vi "AWG simple.vi"() -> ()   [LabVIEW 2015]
uses:
  <instrlib>/niFgen/niFgen.llb/niFgen Output Mode.ctl
  <instrlib>/niFgen/niFgen.llb/niFgen Create Waveform (WDT).vi
panel:
  in  "FGEN Gain":dbl=5.0
  in  "User Gain":dbl=10.0
  out "Sample Rate":dbl
  out "error out":errorcluster
  in  "Resource Name":refnum<k15>="ArbWaveformGen"
  in  "Load Saved Waveform":bool
  in  "Save Current Waveform":bool
  in  "Apply Changes":bool
  in  "stop":bool
  out "Waveform Chart 2":waveform(dbl)(graph)
  out "delta-T":dbl
  in  "Bytes/Sample":dbl=2.0
  out "Rare Samples":dbl
  out "Stable Samples":dbl
  out "Rare Window (ms)":dbl
  in  "Stable window (ms)":dbl=0.1
  out "Waveform File Size (MB)":dbl
  out "Waveform Period (ms)":dbl
  in  "Waveform Samples":dbl
  in  "Bounce Field Frequency (Hz)":dbl=10.0
  in  "Rare":sgl(slide) min=0 max=10 step=0.001 scale=0.0..10.0
  in  "Stable":sgl(slide) min=0 max=10 step=0.001 scale=0.0..10.0
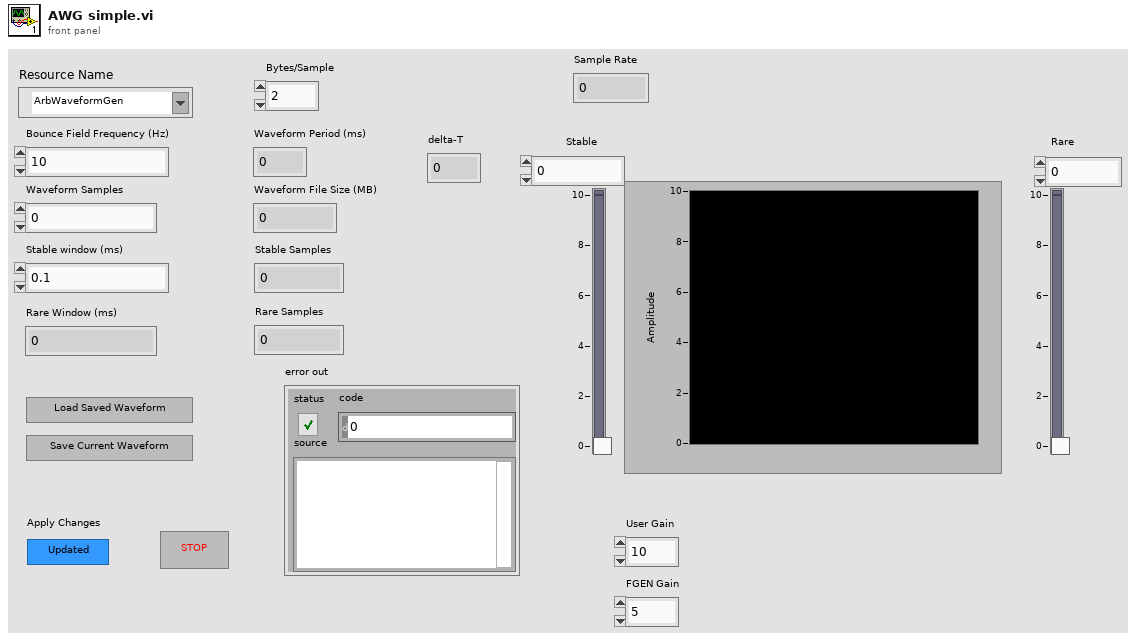
[diagram p1: front panel]
types:
  T1 = typedef "niFgen Output Mode.ctl" = u32
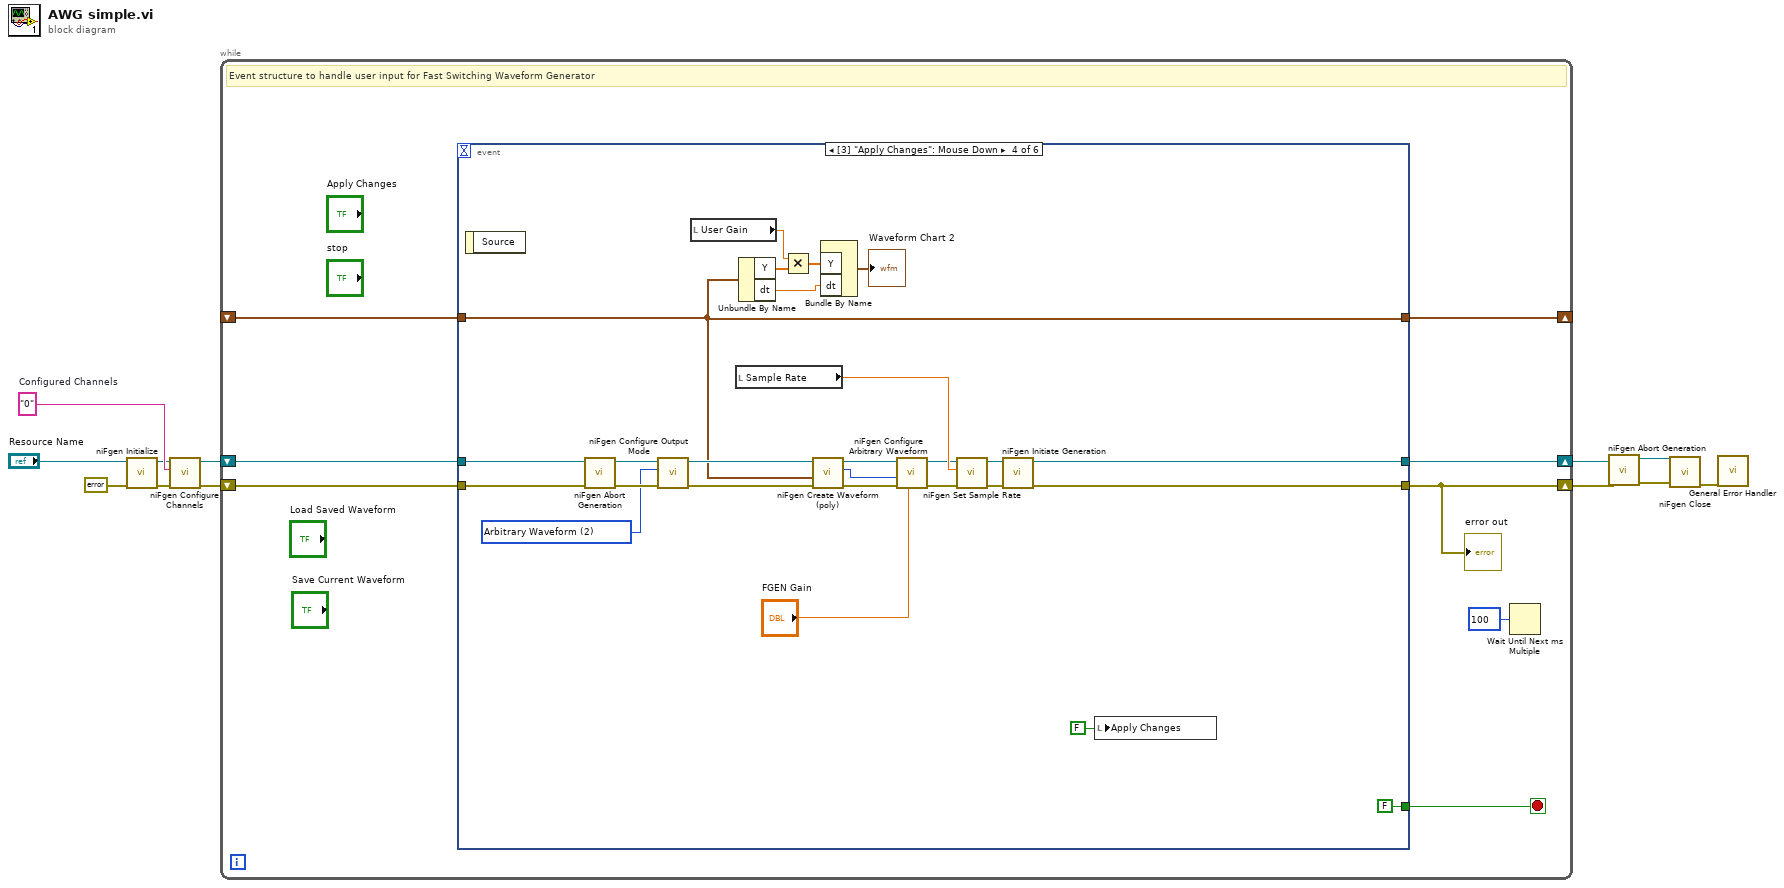
[diagram p0: block diagram]
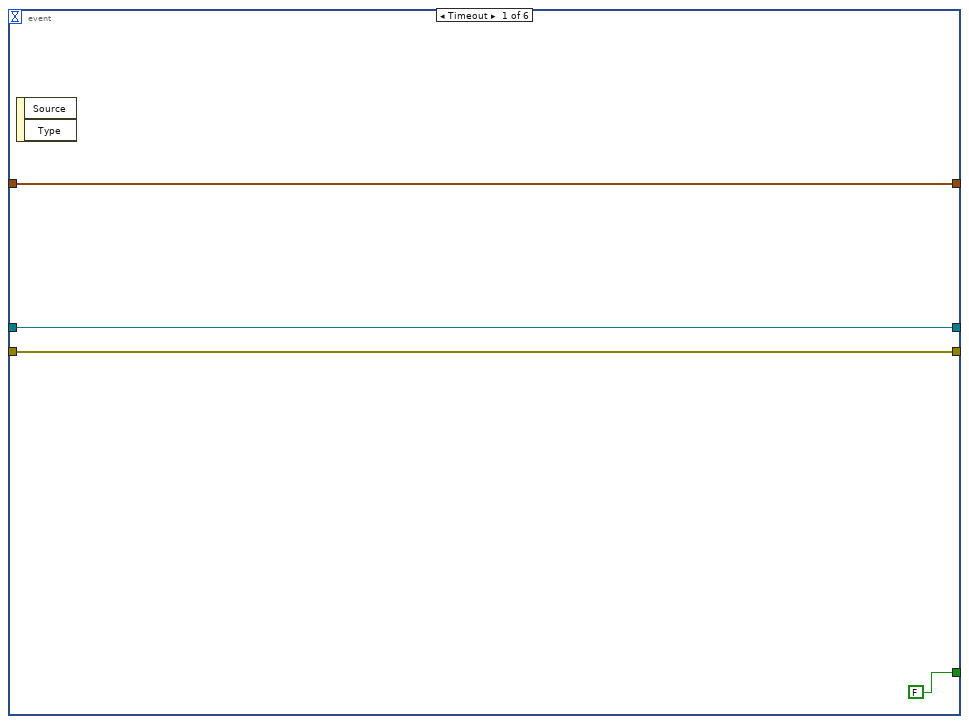
[diagram p2: hidden frame]
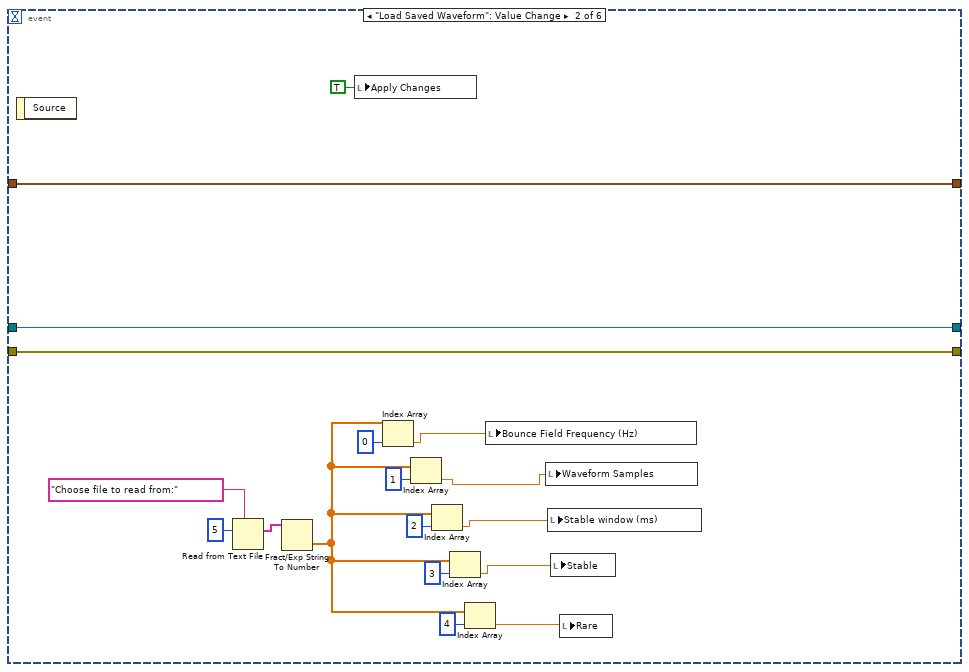
[diagram p3: hidden frame]
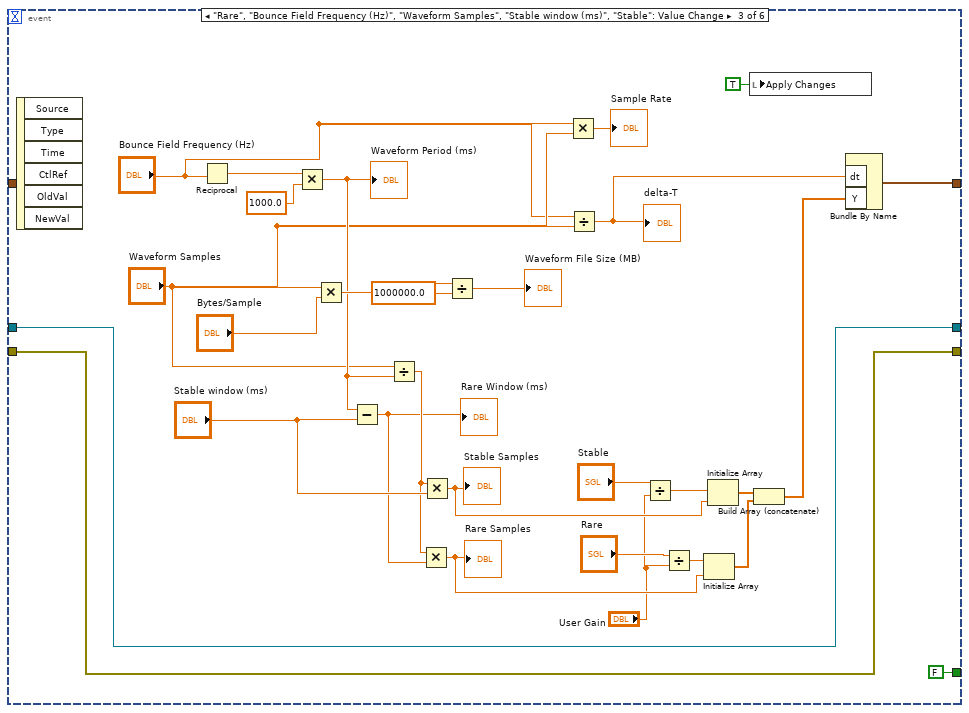
[diagram p4: hidden frame]
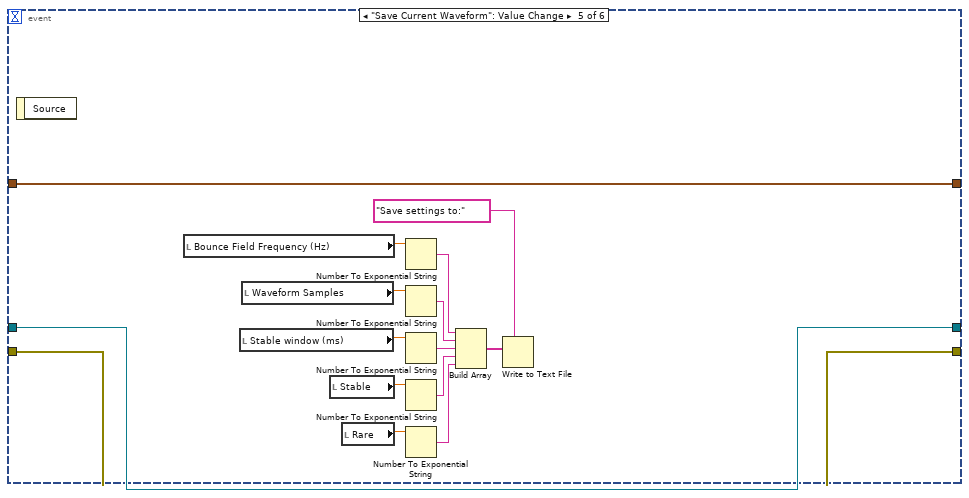
[diagram p5: hidden frame]
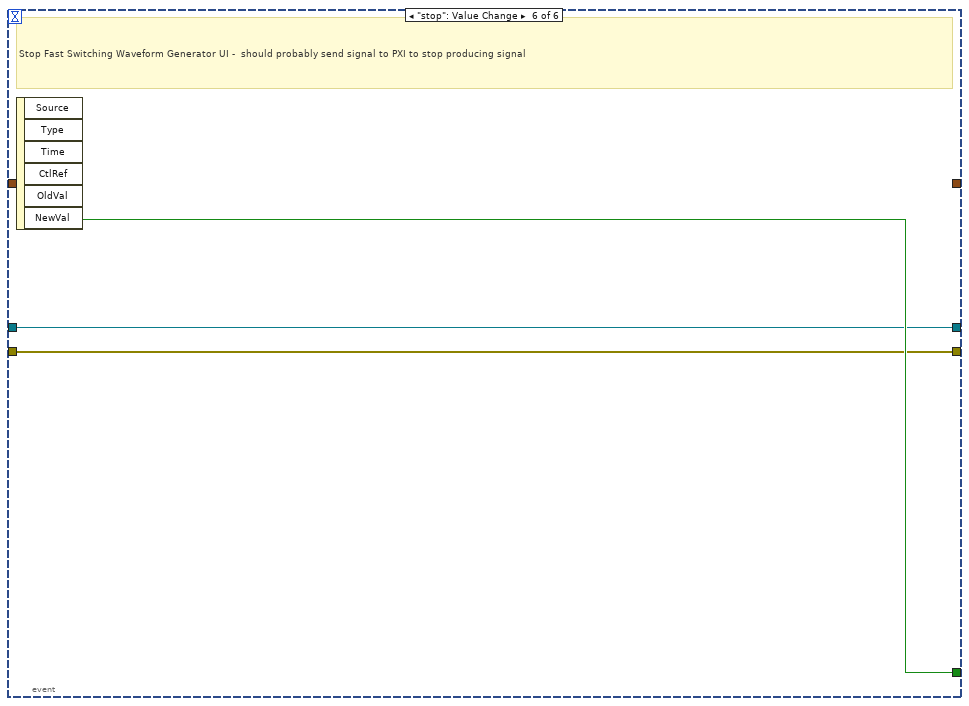
[diagram p6: hidden frame]
diagram:
  w11 = "0"  # Configured Channels
  n1 = call <instrlib>:"niFgen Initialize.vi"("error in (no error)"=errorcluster {"status"=FALSE, "code"=0, "source"=""}, "Resource Name"="Resource Name") -> ("error out"=w10:errorcluster, "Instrument Handle Out"=w9:refnum<k15>)  [unwired: 8 in]
  n2 = call <instrlib>:"niFgen Configure Channels.vi"("error in (no error)"=w10, "Channels"=w11, "Instrument Handle"=w9) -> ("error out"=w5:errorcluster, "Instrument Handle Out"=w6:refnum<k15>)  [unwired: 7 in]
  n3 = while {
    shift-right: [w20] -> _
    shift-left: _ -> [w19]
    shift-right: [w13] -> w4
    shift-left: w6 -> [w15]
    shift-right: [w14] -> w3
    shift-left: w5 -> [w16]
    stop <- w17 stop-if-true
    # "Event structure to handle user input for Fast Switching Waveform Generator"
    n4 = event shown="[3] \"Apply Changes\": Mouse Down" {
      selector: _ -> [_ _ _ _ _ _]
      dyn-events: _ -> [_ _ _ _ _ _]
      timeout: _ -> [_ _ _ _ _ _]
      tunnel: [w24 w27 w56 w77 w112 _] -> w20
      tunnel: w19 -> [w24 w27 _ w77 w112 _]
      tunnel: [FALSE ("NewVal") _ FALSE ("stop") FALSE ("stop") _ w115] -> w17
      tunnel: w16 -> [w21 w25 w53 w81 w99 w114]
      tunnel: w15 -> [w22 w26 w52 w82 w98 w113]
      tunnel: [w21 w25 w53 w95 w99 w114] -> w14
      tunnel: [w22 w26 w52 w94 w98 w113] -> w13
      event Timeout {
        n5 = event-data() -> ()  [unwired: 1 in, 2 out]
      }
      event "Load Saved Waveform": Value Change {
        n6 = event-data() -> ()  [unwired: 1 in, 1 out]
        n7 = Read from Text File(prompt (Open existing file)="Choose file to read from:", count=5) -> (text=w40:string[])  [unwired: 2 in, 3 out]
        n8 = Fract/Exp String To Number(string=w40) -> (number=w33:dbl[])  [unwired: 3 in, 1 out]
        n9 = local write "Apply Changes"(TRUE ("Apply Changes")) -> ()
        n10 = Index Array(array=w33, index=0) -> (element=w38:dbl)
        n11 = Index Array(array=w33, index=1) -> (element=w34:dbl)
        n12 = Index Array(array=w33, index=2) -> (element=w35:dbl)
        n13 = Index Array(array=w33, index=3) -> (element=w36:dbl)
        n14 = Index Array(array=w33, index=4) -> (element=w37:dbl)
        n15 = local write "Bounce Field Frequency (Hz)"(w38) -> ()
        n16 = local write "Waveform Samples"(w34) -> ()
        n17 = local write "Stable window (ms)"(w35) -> ()
        n18 = local write "Stable"(w36) -> ()
        n19 = local write "Rare"(w37) -> ()
      }
      event "Rare", "Bounce Field Frequency (Hz)", "Waveform Samples", "Stable window (ms)", "Stable": Value Change {
        n20 = event-data() -> ()  [unwired: 1 in, 6 out]
        n21 = Reciprocal(x="Bounce Field Frequency (Hz)") -> (1/x=w51:dbl)
        n22 = Multiply(x=w51, y=1000.0) -> (x*y=w59:dbl)
        "Waveform Period (ms)" <- w59
        n23 = Multiply(x="Waveform Samples", y="Bytes/Sample") -> (x*y=w66:dbl)
        n24 = Subtract(x=w59, y="Stable window (ms)") -> (x-y=w68:dbl)
        "Rare Window (ms)" <- w68
        n25 = Divide(x="Waveform Samples", y=w59) -> (x/y=w69:dbl)
        n26 = Multiply(x=w69, y=w68) -> (x*y=w62:dbl)
        "Rare Samples" <- w62
        n27 = Multiply(x=w69, y="Stable window (ms)") -> (x*y=w63:dbl)
        "Stable Samples" <- w63
        n28 = Divide(x=w66, y=1000000.0) -> (x/y=→"Waveform File Size (MB)":dbl)
        n29 = Multiply(x="Bounce Field Frequency (Hz)", y="Waveform Samples") -> (x*y=→"Sample Rate":dbl)
        n30 = Divide(x="Bounce Field Frequency (Hz)", y="Waveform Samples") -> (x/y=w57:dbl)
        "delta-T" <- w57
        n31 = Divide(x="Stable", y="User Gain") -> (x/y=w48:dbl)
        n32 = Divide(x="Rare", y="User Gain") -> (x/y=w46:dbl)
        n33 = Initialize Array(w46, w62) -> (w60:dbl[])
        n34 = Initialize Array(w48, w63) -> (w61:dbl[])
        n35 = local write "Apply Changes"(TRUE ("Apply Changes")) -> ()
        n36 = Build Array (concatenate)(w61, w60) -> (w58:dbl[])
        n37 = Bundle By Name("dt"=w57, "Y"=w58) -> (w56:waveform(dbl))  [unwired: 1 in]
      }
      event "Apply Changes": Mouse Down {
        w83 = T1 2 items=["Standard Function", "Frequency List", "Arbitrary Waveform", "Arbitrary Sequence", "Script"] ("Output Mode (default: 0=Standard Function)")
        n38 = event-data() -> ()  [unwired: 1 in, 1 out]
        n39 = call <instrlib>:"niFgen Abort Generation.vi"("error in (no error)"=w81, "Instrument Handle"=w82) -> ("error out"=w84:errorcluster, "Instrument Handle Out"=w85:refnum<k15>)  [unwired: 8 in]
        n40 = call <instrlib>:"niFgen Configure Output Mode.vi"("error in (no error)"=w84, "Output Mode (default: 0=Standard Function)"=w83, "Instrument Handle"=w85) -> ("error out"=w79:errorcluster, "Instrument Handle Out"=w80:refnum<k15>)  [unwired: 6 in]
        n41 = local read "User Gain"() -> (w73:dbl)
        n42 = local read "Sample Rate"() -> (w90:dbl)
        n43 = Unbundle By Name(w77) -> ("Y"=w74:dbl[], "dt"=w76:dbl)
        n44 = Multiply(x=w73, y=w74) -> (x*y=w75:dbl[])
        n45 = call-poly <instrlib>:"niFgen Create Waveform (poly).vi"("error in (no error)"=w79, "Waveform"=w77, "Instrument Handle"=w80) -> ("error out"=w86:errorcluster, "Waveform Handle"=w88:i32, "Instrument Handle Out"=w93:refnum<k15>)  [unwired: 6 in]
        n46 = Bundle By Name("Y"=w75, "dt"=w76) -> (→"Waveform Chart 2":waveform(dbl))  [unwired: 1 in]
        n47 = call <instrlib>:"niFgen Configure Arbitrary Waveform.vi"("Gain"="FGEN Gain", "error in (no error)"=w86, "Waveform Handle"=w88, "Instrument Handle"=w93) -> ("error out"=w87:errorcluster, "Instrument Handle Out"=w89:refnum<k15>)  [unwired: 6 in]
        n48 = call <instrlib>:"niFgen Set Sample Rate.vi"("error in (no error)"=w87, "Sample Rate (Samp/s)"=w90, "Instrument Handle"=w89) -> ("error out"=w91:errorcluster, "Instrument Handle Out"=w92:refnum<k15>)  [unwired: 7 in]
        n49 = call <instrlib>:"niFgen Initiate Generation.vi"("error in (no error)"=w91, "Instrument Handle"=w92) -> ("error out"=w95:errorcluster, "Instrument Handle Out"=w94:refnum<k15>)  [unwired: 8 in]
        n50 = local write "Apply Changes"(FALSE ("Apply Changes")) -> ()
      }
      event "Save Current Waveform": Value Change {
        n51 = event-data() -> ()  [unwired: 1 in, 1 out]
        n52 = local read "Bounce Field Frequency (Hz)"() -> (w111:dbl)
        n53 = local read "Stable window (ms)"() -> (w107:dbl)
        n54 = local read "Waveform Samples"() -> (w108:dbl)
        n55 = local read "Stable"() -> (w110:sgl)
        n56 = local read "Rare"() -> (w109:sgl)
        n57 = Number To Exponential String(number=w111) -> (E-format string=w106:string)  [unwired: 3 in]
        n58 = Number To Exponential String(number=w108) -> (E-format string=w103:string)  [unwired: 3 in]
        n59 = Number To Exponential String(number=w107) -> (E-format string=w102:string)  [unwired: 3 in]
        n60 = Number To Exponential String(number=w110) -> (E-format string=w101:string)  [unwired: 3 in]
        n61 = Number To Exponential String(number=w109) -> (E-format string=w100:string)  [unwired: 3 in]
        n62 = Build Array(w106, w103, w102, w101, w100) -> (w105:string[])
        n63 = Write to Text File(prompt (Choose or enter file path)="Save settings to:", text=w105) -> ()  [unwired: 2 in, 3 out]
      }
      event "stop": Value Change {
        # "Stop Fast Switching Waveform Generator UI -  should probably send signal to PXI to stop producing signal"
        n64 = event-data() -> ("NewVal"=w115:bool)  [unwired: 1 in, 5 out]
      }
    }
    "error out" <- w14
    n65 = Wait Until Next ms Multiple(millisecond multiple=u32 100) -> ()  [unwired: 1 out]
  }
  n66 = call <instrlib>:"niFgen Abort Generation.vi"("error in (no error)"=w3, "Instrument Handle"=w4) -> ("error out"=w2:errorcluster, "Instrument Handle Out"=w1:refnum<k15>)  [unwired: 8 in]
  n67 = call <instrlib>:"niFgen Close.vi"("error in (no error)"=w2, "Instrument Handle"=w1) -> ("error out"=w8:errorcluster)  [unwired: 9 in]
  n68 = call <vilib>:"General Error Handler.vi"("error in (no error)"=w8) -> ()  [unwired: 10 in, 5 out]
